vi "PCIe Signal Routing.vi"(6 "trigger master index":i32, 8 "error in":errorcluster, 9 "sync pulse rtsi line":string="RTSI1", 10 "start trigger rtsi line":string="RTSI0", 11 "fpga interfaces in":refnum<k20>[](array[refnum])) -> (0 "error out":errorcluster, 3 "fpga interfaces out":refnum<k20>[](array[refnum]))   [LabVIEW 2018, in "GettingStarted_5785_Host.lvlib"]
uses:
  GettingStarted_5785_Host.lvlib
  <instrlib>/FlexRIO/API/Host/v1/NI FlexRIO/API/Get Property Reference - Fpga Small.vi
  <resource>/objmgr/niflexrioapi.rc
  <instrlib>/FlexRIO/API/Host/v1/NI FlexRIO API v1.lvlib
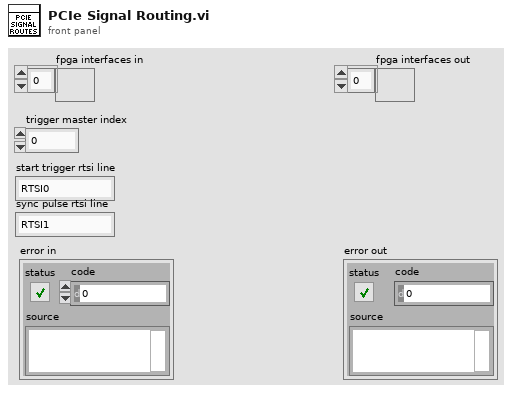
[diagram p1: front panel]
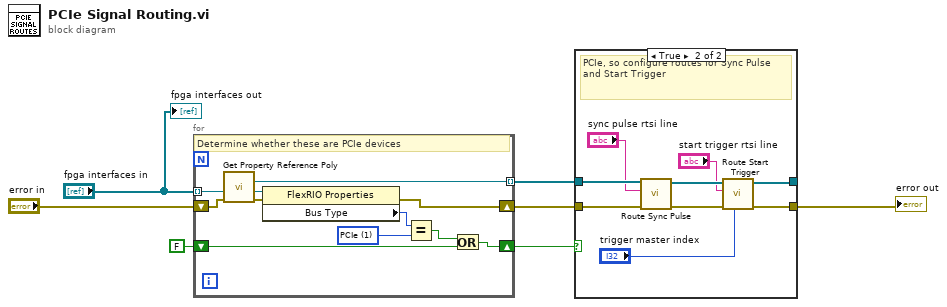
[diagram p0: block diagram]
diagram:
  n1 = for {
    tunnel: [w14] -> w7 mode=indexing
    shift-right: [w12] -> w6
    shift-left: "error in" -> [w13]
    tunnel: "fpga interfaces in" -> [w11] mode=indexing
    shift-right: [w10] -> w2
    shift-left: FALSE -> [w9]
    w16 = 1 items=["PXIe", "PCIe"] ("Description:Bus Type")
    # "Determine whether these are PCIe devices"
    n2 = call-poly <instrlib>:"Get Property Reference Poly.vi"("error in (no error)"=w13, "fpga interface in"=w11) -> ("error out"=w17:errorcluster, "property reference"=w18:refnum<k20>, "fpga interface out"=w14:refnum<k20>)  [unwired: 4 in]
    n3 = property class="FlexRIO Properties"(reference=w18, error in=w17) -> (error out=w12:errorcluster, "Bus Type"=w15:i32)  [unwired: 1 out]
    n4 = Equal?(x=w15, y=w16) -> (x = y?=w8:bool)
    n5 = Or(x=w8, y=w9) -> (x .or. y?=w10:bool)
  }
  n6 = case shown="True" w2 {
    tunnel: [w19 w24] -> w5
    tunnel: [w20 w25] -> _
    tunnel: w7 -> [w20 w28]
    tunnel: w6 -> [w19 w29]
    frame False {
      # "Not PCIe, manual routing is not necessary"
    }
    frame True {
      # "PCIe, so configure routes for Sync Pulse and Start Trigger"
      n7 = call "Route Sync Pulse.vi"("error in"=w29, "sync pulse rtsi line"="sync pulse rtsi line", "fpga interfaces in"=w28) -> ("error out"=w27:errorcluster, "fpga interfaces out"=w26:refnum<k20>[])  [unwired: 7 in]
      n8 = call "Route Start Trigger.vi"("trigger master index"="trigger master index", "error in"=w27, "start trigger rtsi line"="start trigger rtsi line", "fpga interfaces in"=w26) -> ("error out"=w24:errorcluster, "fpga interfaces out"=w25:refnum<k20>[])  [unwired: 6 in]
    }
  }
  "error out" <- w5
  "fpga interfaces out" <- "fpga interfaces in"
